vi "TEMPDo.vi"(8 "error in (no error)":errorcluster, 10 "Actor in":refnum<class "Actor.lvclass">, 11 "DNL_Message Template":refnum<class "Message.lvclass">) -> (0 "error out":errorcluster, 2 "Actor out":refnum<class "Actor.lvclass">)   [LabVIEW 2015, in "PV Message Template.lvclass"]
doc: "This VI delivers the message to the actor by calling the appropriate method(s) on the actor."
uses:
  PV Message Template.lvclass
  <vilib>/ActorFramework/Actor/Actor.lvclass
  <vilib>/ActorFramework/Message/Message.lvclass
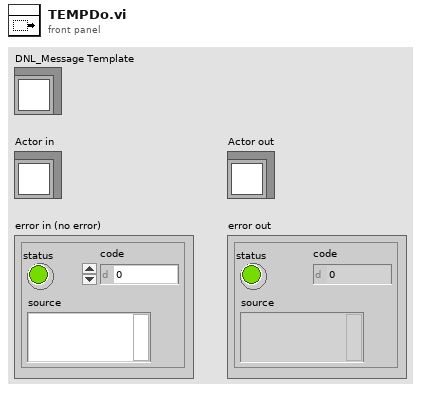
[diagram p1: front panel]
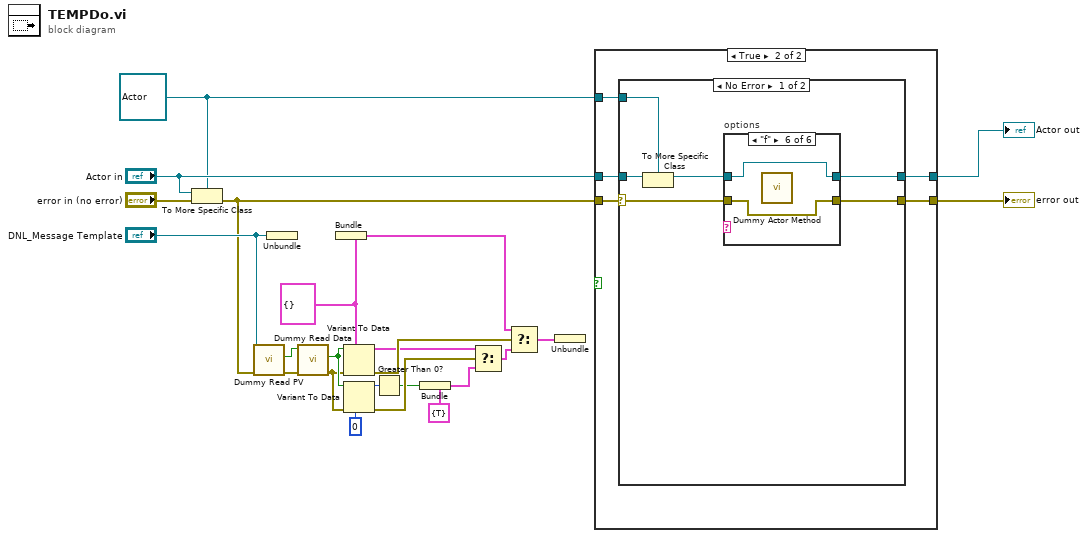
[diagram p0: block diagram]
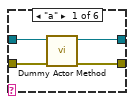
[diagram p3: hidden frame]
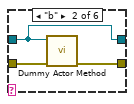
[diagram p4: hidden frame]
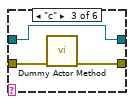
[diagram p5: hidden frame]
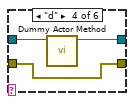
[diagram p6: hidden frame]
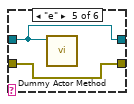
[diagram p7: hidden frame]
diagram:
  w13 = cluster{} {} ("Type")
  w19 = refnum<class "Actor.lvclass"> refnum ("Actor in")
  n1 = To More Specific Class(target class=w19, reference="Actor in", error in="error in (no error)") -> (error out=w17:errorcluster)  [unwired: 1 out]
  n2 = call "Dummy Read PV.vi"("error in (no error)"=w17, "Actor in"="DNL_Message Template") -> ("error out"=w16:errorcluster, "Boolean"=w12:bool)  [unwired: 7 in, 1 out]
  n3 = Unbundle ("Pre-Unbundler")("DNL_Message Template") -> ()  [unwired: 1 out]
  n4 = call "Dummy Read Data.vi"("error in (no error)"=w16, "Actor in"=w12) -> ("error out"=w9:errorcluster, "Boolean"=w10:bool)  [unwired: 7 in, 1 out]
  n5 = Bundle ("Pre-Bundler")(cluster=w13) -> (w14:cluster{void})  [unwired: 1 in]
  n6 = Variant To Data(error in=w9, type=w13, Variant=w10) -> (data=w6:cluster{}, error out=w15:errorcluster)
  n7 = Variant To Data ("I16-Conversion")(error in=w9, type=i16 0 ("I16-Conversion-Constant"), Variant=w10) -> (data=w4:i16, error out=w7:errorcluster)
  n8 = Greater Than 0? ("I16-Comp0")(x=w4) -> (x > 0?=w2:bool)
  n9 = Bundle ("I16-Bundle")(cluster=cluster{bool} {TRUE} ("I16-Cluster"), w2) -> (w1:cluster{bool})
  n10 = Select ("I16-Select")(t=w6, s=w7, f=w1) -> (s? t:f=w5:cluster{bool})
  n11 = Select ("MainSelect")(t=w14, s=w15, f=w5) -> (s? t:f=w8:cluster{bool})
  n12 = Unbundle ("Main-Unbundler")(w8) -> ()  [unwired: 1 out]
  n13 = case "Execute?" shown="True" {
    selector: _ -> [_ _]
    tunnel: [w24 w30] -> w22
    tunnel: [w25 w29] -> w21
    tunnel: "Actor in" -> [w25 w28]
    tunnel: w19 -> [_ w27]
    tunnel: w17 -> [w24 w26]
    frame False {
    }
    frame True {
      n14 = case shown="No Error" w26 {
        selector: w26 -> [w34 w55]
        tunnel: [w36 w55] -> w30
        tunnel: [w35 w54] -> w29
        tunnel: w28 -> [w33 w54]
        tunnel: w27 -> [w32 _]
        frame No Error {
          n15 = To More Specific Class(target class=w32, reference=w33) -> (specific class reference=w31:refnum<class "Actor.lvclass">)  [unwired: 1 in, 1 out]
          n16 = case "options" shown="\"f\"" {
            selector: _ -> [_ _ _ _ _ _]
            tunnel: [w40 w43 w46 w49 w50 w52] -> w36
            tunnel: [w39 w41 w44 w47 w51 w53] -> w35
            tunnel: w34 -> [w38 w42 w45 w49 w50 w52]
            tunnel: w31 -> [w37 w41 w44 w48 w51 w53]
            frame "a" {
              n17 = call "Dummy Actor Method.vi"("error in (no error)"=w38, "Actor in"=w37) -> ("error out"=w40:errorcluster, "Actor out"=w39:refnum<class "Actor.lvclass">)  [unwired: 8 in]
            }
            frame "b" {
              n18 = call "Dummy Actor Method.vi"("error in (no error)"=w42, "Actor in"=w41) -> ("error out"=w43:errorcluster)  [unwired: 8 in, 1 out]
            }
            frame "c" {
              n19 = call "Dummy Actor Method.vi"("error in (no error)"=w45) -> ("error out"=w46:errorcluster)  [unwired: 9 in, 1 out]
            }
            frame "d" {
              n20 = call "Dummy Actor Method.vi"("Actor in"=w48) -> ("Actor out"=w47:refnum<class "Actor.lvclass">)  [unwired: 9 in, 1 out]
            }
            frame "e" {
              n21 = call "Dummy Actor Method.vi"("Actor in"=w51) -> ()  [unwired: 9 in, 2 out]
            }
            frame "f" {
              n22 = call "Dummy Actor Method.vi"() -> ()  [unwired: 10 in, 2 out]
            }
          }
        }
        frame Error {
        }
      }
    }
  }
  "error out" <- w22
  "Actor out" <- w21
